vi "Conversion.vi"(5 "number_repetitions":i32, 7 "q_samples":i32=50, 9 "triggers":u32[](array[numeric]), 10 "timetags":u32[](graph), 11 "Rabi_parameters":T1) -> (1 "triggers":u32[][](array[numeric]), 3 "timetags":u32[][](array[numeric]))   [LabVIEW 2018]
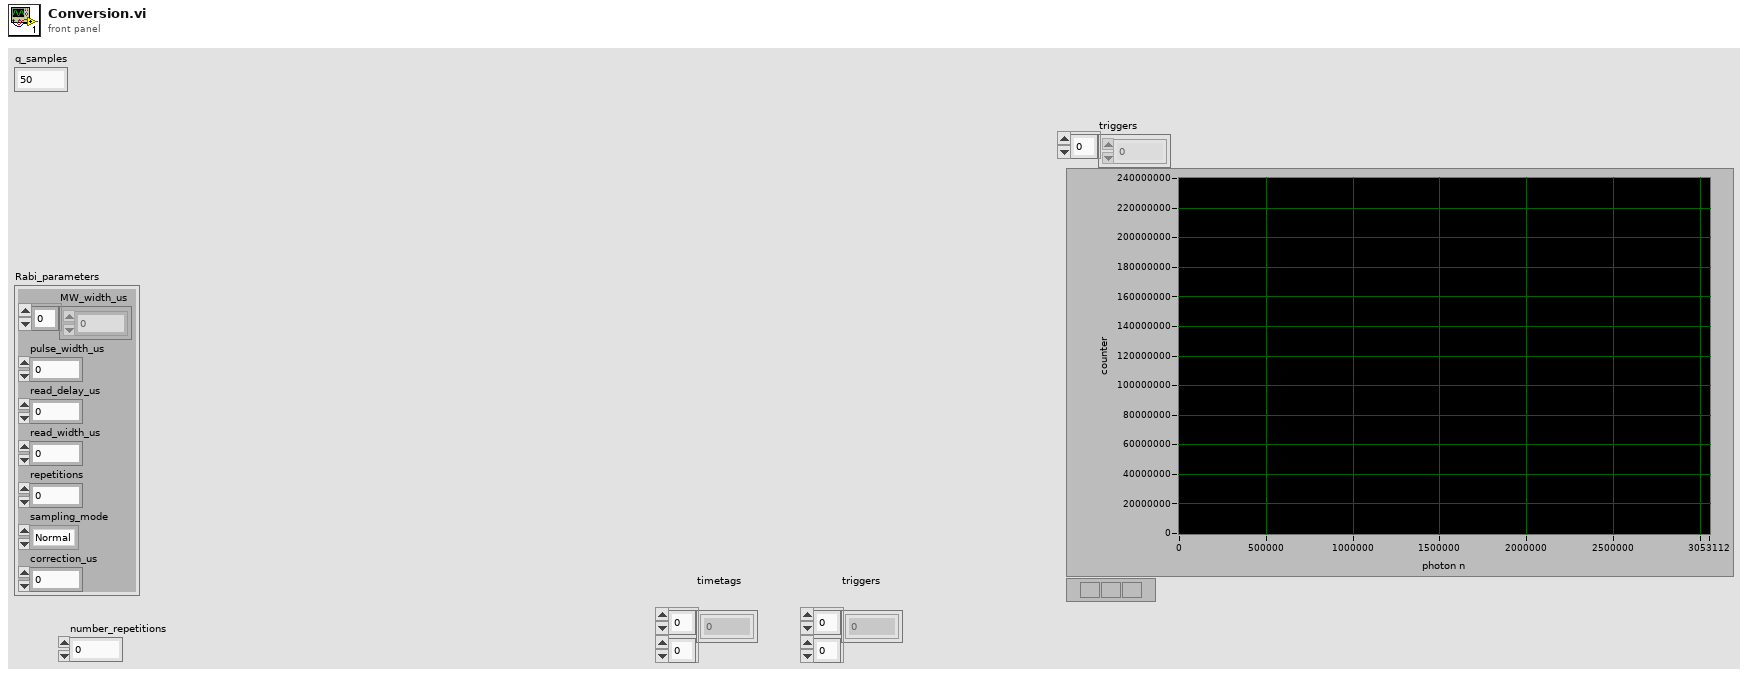
[diagram p1: front panel]
types:
  T1 = cluster{"MW_width_us":dbl[], "pulse_width_us":dbl, "read_delay_us":dbl, "read_width_us":dbl, "repetitions":i32, "sampling_mode":enum16{"Normal", "Sweep"}, "correction_us":dbl}
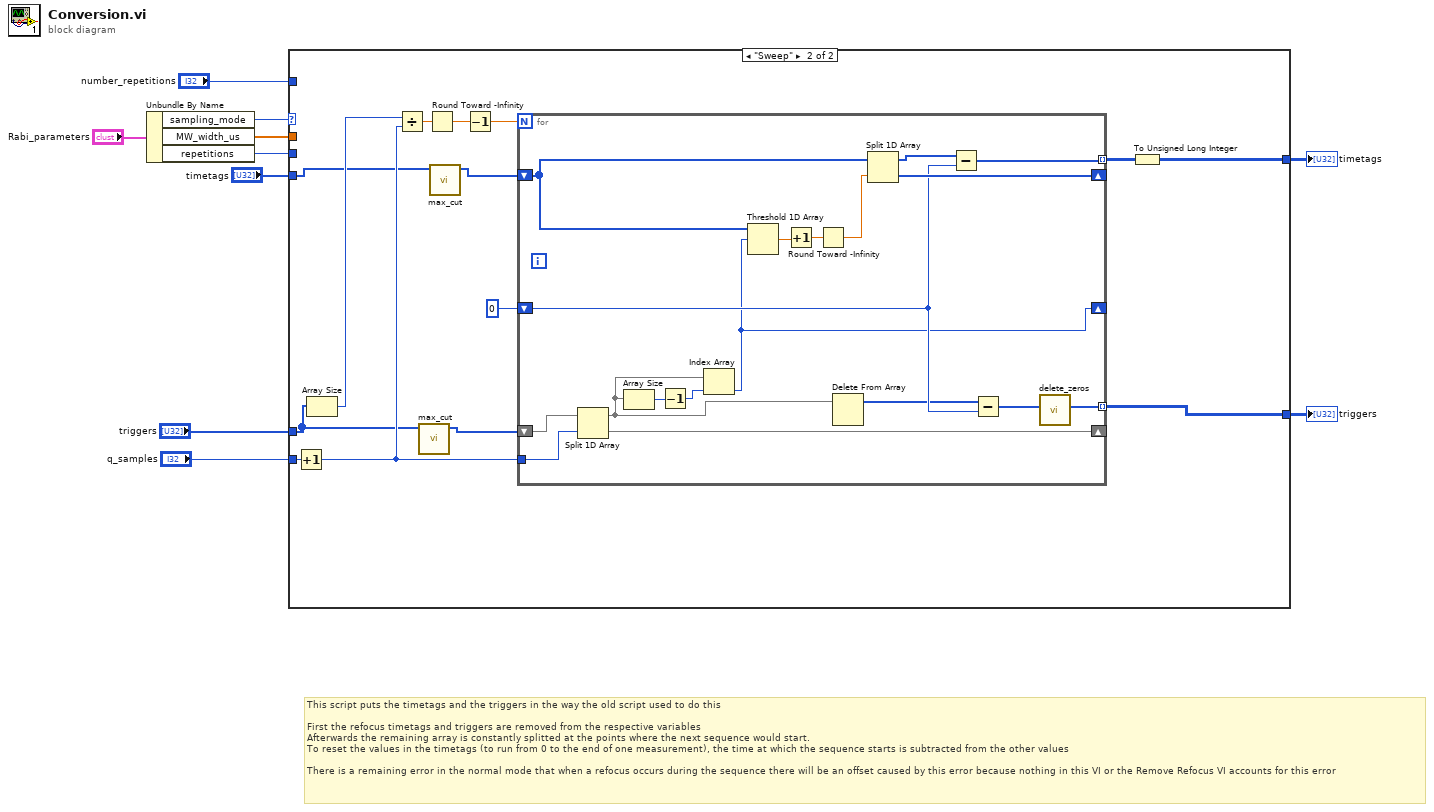
[diagram p0: block diagram]
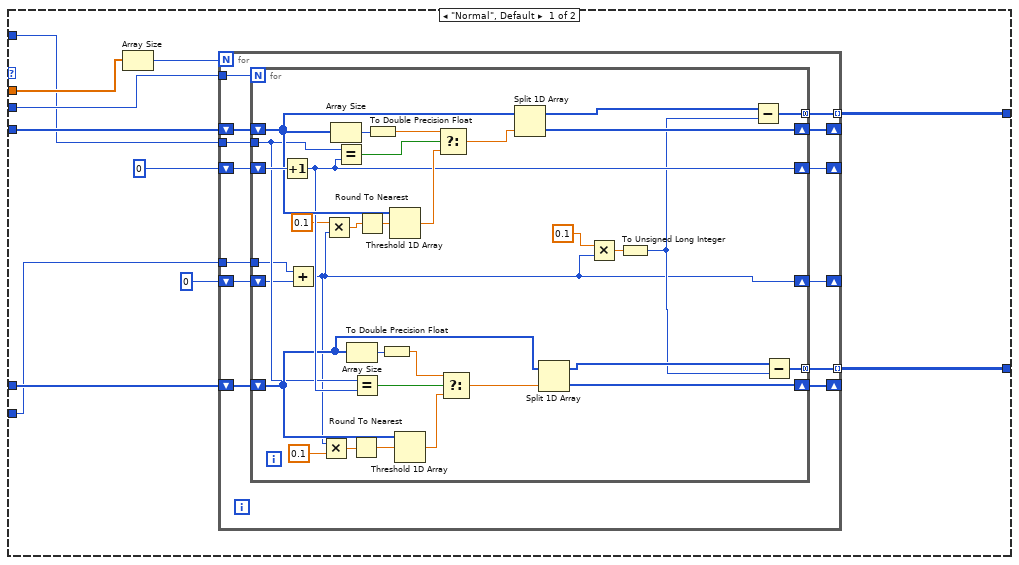
[diagram p2: hidden frame]
diagram:
  # "This script puts the timetags and the triggers in the way the old script used to do this\n\nFirst the refocus timetags and triggers are removed from the respective variables\nAfterwards the remaining array is constantly splitted at the points where the next sequence would start.\nTo reset the values in the timetags (to run from 0 to the end of one measurement), the time at which the sequence starts is subtracted from the other values\n\nThere is a remaining error in the normal mode that when a refocus occurs during the sequence there will be an offset caused by this error because nothing in this VI or the Remove Refocus VI accounts for this error"
  n1 = Unbundle By Name("Rabi_parameters") -> ("sampling_mode"=w9:enum16{"Normal", "Sweep"}, "MW_width_us"=w6:dbl[], "repetitions"=w5:i32)
  n2 = case shown="\"Sweep\"" w9 {
    tunnel: "timetags" -> [w19 w70]
    tunnel: "triggers" -> [w17 w73]
    tunnel: [w16 w80] -> w7
    tunnel: [w18 w68] -> w8
    tunnel: w6 -> [w21 _]
    tunnel: w5 -> [w20 _]
    tunnel: "number_repetitions" -> [w13 _]
    tunnel: "q_samples" -> [w11 w77]
    frame "Normal", Default {
      n3 = Array Size(array=w21) -> (size(s)=w15:i32)
      n4 = for {
        N: w15 -> [_]
        tunnel: w20 -> [w34]
        shift-right: [w33] -> _
        shift-left: u32 0 -> [w26]
        shift-right: [w31] -> _
        shift-left: w19 -> [w32]
        tunnel: [w30] -> w18 mode=indexing
        shift-right: [w27] -> _
        shift-left: w17 -> [w29]
        tunnel: [w28] -> w16 mode=indexing
        tunnel: w13 -> [w25]
        shift-right: [w22] -> _
        shift-left: u32 0 -> [w24]
        tunnel: w11 -> [w23]
        n5 = for {
          N: w34 -> [_]
          shift-right: [w58] -> w33
          shift-left: w26 -> [w67]
          shift-right: [w50] -> w31
          shift-left: w32 -> [w61]
          tunnel: [w48] -> w30 mode=concatenating
          shift-right: [w53] -> w27
          shift-left: w29 -> [w55]
          tunnel: [w51] -> w28 mode=concatenating
          tunnel: w25 -> [w47]
          shift-right: [w35] -> w22
          shift-left: w24 -> [w43]
          tunnel: w23 -> [w44]
          n6 = Increment(x=w67) -> (x+1=w58:u32)
          n7 = Add(x=w44, y=w43) -> (x+y=w35:u32)
          n8 = Multiply(x=w35, y=0.1 ("x")) -> (x*y=w40:dbl)
          n9 = Multiply(x=0.1, y=w35) -> (x*y=w41:dbl)
          n10 = Array Size(array=w61) -> (size(s)=w63:i32)
          n11 = Equal?(x=w47, y=w58) -> (x = y?=w66:bool)
          n12 = Array Size(array=w55) -> (size(s)=w60:i32)
          n13 = Round To Nearest(number=w40) -> (nearest integer value=w45:dbl)
          n14 = Equal?(x=w47, y=w58) -> (x = y?=w54:bool)
          n15 = Round To Nearest(number=w41) -> (nearest integer value=w46:dbl)
          n16 = To Double Precision Float(number=w63) -> (double precision float=w64:dbl)
          n17 = To Double Precision Float(number=w60) -> (double precision float=w59:dbl)
          n18 = Threshold 1D Array(2:w46, 3:w61) -> (0:w65:dbl)  [unwired: 1 in]
          n19 = Threshold 1D Array(2:w45, 3:w55) -> (0:w57:dbl)  [unwired: 1 in]
          n20 = Select(t=w64, s=w66, f=w65) -> (s? t:f=w62:dbl)
          n21 = Select(t=w59, s=w54, f=w57) -> (s? t:f=w56:dbl)
          n22 = Split 1D Array(array=w61, index=w62) -> (first subarray=w49:u32[], second subarray=w50:u32[])
          n23 = Split 1D Array(array=w55, index=w56) -> (first subarray=w52:u32[], second subarray=w53:u32[])
          n24 = Multiply(x=0.1, y=w35) -> (x*y=w38:dbl)
          n25 = To Unsigned Long Integer(number=w38) -> (unsigned 32bit integer=w37:u32)
          n26 = Subtract(x=w49, y=w37) -> (x-y=w48:u32[])
          n27 = Subtract(x=w52, y=w37) -> (x-y=w51:u32[])
        }
      }
    }
    frame "Sweep" {
      n28 = Increment(x=w77) -> (x+1=w76:i32)
      n29 = Array Size(array=w73) -> (size(s)=w78:i32)
      n30 = Divide(x=w78, y=w76) -> (x/y=w79:dbl)
      n31 = call "max_cut.vi"("triggers_in"=w73) -> ("fixed"=w72:u64[])  [unwired: 10 in]
      n32 = Round Toward -Infinity(1:w79) -> (0:w75:dbl)
      n33 = call "max_cut.vi"("triggers_in"=w70) -> ("fixed"=w71:u64[])  [unwired: 10 in]
      n34 = Decrement(x=w75) -> (x-1=w74:dbl)
      n35 = for {
        N: w74 -> [_]
        tunnel: [w97] -> w69 mode=indexing
        shift-right: [w99] -> _
        shift-left: w71 -> [w88]
        shift-right: [w94] -> _
        shift-left: w72 -> [w95]
        tunnel: w76 -> [w96]
        shift-right: [w85] -> _
        shift-left: u64 0 -> [w87]
        tunnel: [w84] -> w80 mode=indexing
        n36 = Split 1D Array(array=w95, index=w96) -> (first subarray=w82:u64[], second subarray=w94:u64[])
        n37 = Array Size(array=w82) -> (size(s)=w93:i32)
        n38 = Decrement(x=w93) -> (x-1=w92:i32)
        n39 = Index Array(array=w82, index=w92) -> (element=w85:u64)
        n40 = Threshold 1D Array(2:w85, 3:w88) -> (0:w91:dbl)  [unwired: 1 in]
        n41 = Increment(x=w91) -> (x+1=w90:dbl)
        n42 = Round Toward -Infinity(1:w90) -> (0:w89:dbl)
        n43 = Delete From Array(array=w82) -> (array with subset deleted=w83:u64[])  [unwired: 2 in, 1 out]
        n44 = Split 1D Array(array=w88, index=w89) -> (first subarray=w98:u64[], second subarray=w99:u64[])
        n45 = Subtract(x=w98, y=w87) -> (x-y=w97:u64[])
        n46 = Subtract(x=w83, y=w87) -> (x-y=w86:u64[])
        n47 = call "delete_zeros.vi"("array_in"=w86) -> ("array_out"=w84:u32[])  [unwired: 10 in]
      }
      n48 = To Unsigned Long Integer(number=w69) -> (unsigned 32bit integer=w68:u32[][])
    }
  }
  "timetags" <- w8
  "triggers" <- w7
